vi "Read Transmission Data Unit.vi"(8 "error in (no error)":errorcluster, 11 "Modbus instance in":refnum<class "Modbus API.lvclass">) -> (0 "error out":errorcluster, 2 "transmission data unit":refnum<class "Transmission Data Unit.lvclass">, 3 "Modbus instance out":refnum<class "Modbus API.lvclass">)   [LabVIEW 2020, in "SubVIs.lvlib" / "Modbus API.lvclass"]
doc: "This VI is an accessor for the transmission data unit stored in the Modbus instance. This accessor can be used as a property node. The transmission data unit is used by the device to determine how to pack and unpack data coming from the physical bus."
uses:
  <vilib>/Modbus/subvis/Modbus API/Modbus API.lvclass
  <vilib>/Modbus/subvis/Transmission Data Unit (ADU)/Transmission Data Unit/Transmission Data Unit.lvclass
  <vilib>/Modbus/subvis/Modbus API/Modbus API.lvclass/Modbus API.ctl
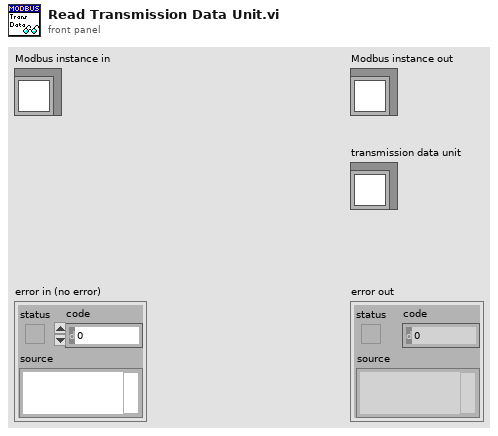
[diagram p1: front panel]
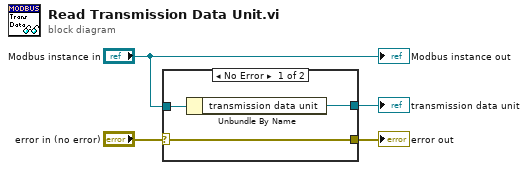
[diagram p0: block diagram]
diagram:
  n1 = case shown="No Error" "error in (no error)" {
    selector: "error in (no error)" -> [w5 w8]
    tunnel: "Modbus instance in" -> [w7 _]
    tunnel: [w6 _] -> w3
    tunnel: [w5 w8] -> w1
    frame No Error {
      n2 = Unbundle By Name(w7) -> ("transmission data unit"=w6:refnum<class "Transmission Data Unit.lvclass">)
    }
    frame Error {
    }
  }
  "error out" <- w1
  "transmission data unit" <- w3
  "Modbus instance out" <- "Modbus instance in"
